vi "Target.vi"() -> ()   [LabVIEW 2025]
uses:
  <vilib>/Platform/TimedLoop/XDataNode/timing_clust.ctl
  <vilib>/Platform/TimedLoop/XDataNode/nitl_modes.ctl
  <vilib>/Platform/TimedLoop/XDataNode/wakeup.ctl
  <vilib>/rvi/Emulation/niFpgaSctlEmulationGetInTimedLoop.vi
  <vilib>/rvi/Emulation/niFpgaEmulationReportErrorSimple.vi
  <vilib>/rvi/Emulation/niFpgaGetClockAttributes.vi
  <vilib>/rvi/Emulation/niFpgaCriticalErrorInLSC.vi
  <vilib>/rvi/linearAlgebra/MatrixMultiply/simVIs/SubVI/nifxpla_MatrixMultiply_SimMatrixSizes.vi
  <vilib>/rvi/linearAlgebra/MatrixMultiply/simVIs/SubVI/nifxpla_MatrixMultiply_Sim4WireAdapterVector.vi
  <vilib>/rvi/linearAlgebra/MatrixMultiply/simVIs/SubVI/nifxpla_MatrixMultiply_SimFrameHandShake.vi
  <vilib>/rvi/linearAlgebra/MatrixMultiply/simVIs/SubVI/nifxpla_MatrixMultiply_SimEndlessCounter.vi
  <vilib>/rvi/linearAlgebra/MatrixMultiply/simVIs/SubVI/nifxpla_MatrixMultiply_SimVectorDataBuffer.vi
  <vilib>/rvi/ClientSDK/Core/DevComputerLib/Private/Multiply(dfxp64).vi
  <vilib>/rvi/ClientSDK/Core/DevComputerLib/Private/Dfxp128ToDfxp256.vi
  <vilib>/rvi/ClientSDK/Core/DevComputerLib/Private/Add(dfxp256).vi
  <vilib>/rvi/ClientSDK/Core/DevComputerLib/Private/Subtract(dfxp256).vi
  <vilib>/rvi/ClientSDK/Core/DevComputerLib/Private/ToDfxp64(dfxp256).vi
  <vilib>/platform/TimedLoop/XDataNode/XDataNode.xnode
  <vilib>/rvi/linearAlgebra/MatrixMultiply/XNode/nifxpla_MatrixMultiply.xnode
  <vilib>/rvi/linearAlgebra/MatrixMultiply/simVIs/nifxpla_MatrixMultiply_SimTemplateEinEout.vi
  <vilib>/rvi/linearAlgebra/MatrixMultiply/simVIs/nifxpla_MatrixMultiply_SimTemplateEinVout.vi
  <vilib>/rvi/linearAlgebra/MatrixMultiply/simVIs/nifxpla_MatrixMultiply_SimTemplateVinEout.vi
  <vilib>/rvi/linearAlgebra/MatrixMultiply/simVIs/nifxpla_MatrixMultiply_SimTemplateVinVout.vi
  <vilib>/Platform/TimedLoop/XDataNode/XDNodeRunTimeDep.lvlib
panel:
  out "C3+B":fxp<+/-,33,17>[](array[numeric])
  out "C3":fxp<+/-,32,16>[](array[numeric])
  out "Cycle Count 3":i32
  out "C2+B":fxp<+/-,33,17>[](array[numeric])
  out "C2":fxp<+/-,32,16>[](array[numeric])
  out "Cycle Count 2":i32
  out "C1+B":fxp<+/-,33,17>[](array[numeric])
  out "C1":fxp<+/-,32,16>[](array[numeric])
  out "Cycle Count":i32
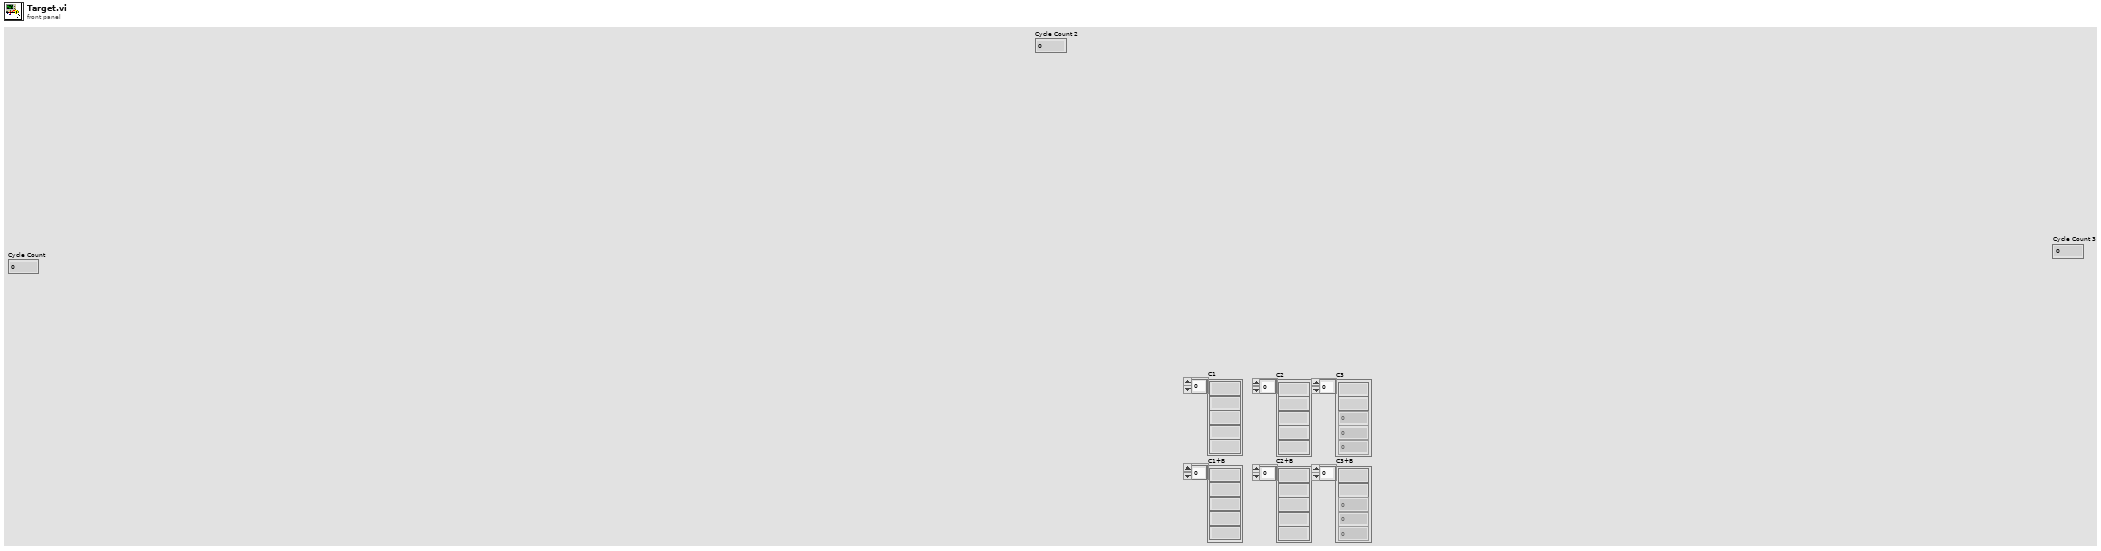
[diagram p1: front panel]
types:
  T1 = typedef "XDNodeRunTimeDep.lvlib/timing_clust.ctl" = cluster{"Expected End [f-1]":u64, "Actual End [f-1]":u64, "Finished Late? [f-1]":bool, "Expected End [i-1]":u64, "Actual End [i-1]":u64, "Finished Late? [i-1]":bool, "Expected Start [i]":u64, "Actual Start [i]":u64, "Expected Start [f]":u64, "Actual Start [f]":u64, "Source Name":string, "Structure Name":string, "Period":i64, "Deadline":i64, "Offset":i64, "Start":i64, "Priority":i32, "Timeout":i32, "Mode":T2, "Wakeup Reason":T3, "Error":errorcluster, "Source Type":string, "Secondary Source Type":string, "Global End Time":u64, "Global Start Time":u64, "Frame Duration":u64, "Iteration Duration":u64, "Assigned CPU":i32, "I/O Scan Engine Mode":u32}
  T2 = typedef "XDNodeRunTimeDep.lvlib/nitl_modes.ctl" = enum32{"No Change", "Process missed periods, maintain original phase", "Discard missed periods, maintain original phase", "Process missed periods, ignore original phase", "Discard missed periods, ignore original phase"}
  T3 = typedef "XDNodeRunTimeDep.lvlib/wakeup.ctl" = enum32{"Normal", "Aborted", "Asynchronous wakeup", "Timing source error", "Timed loop error", "Timeout"}
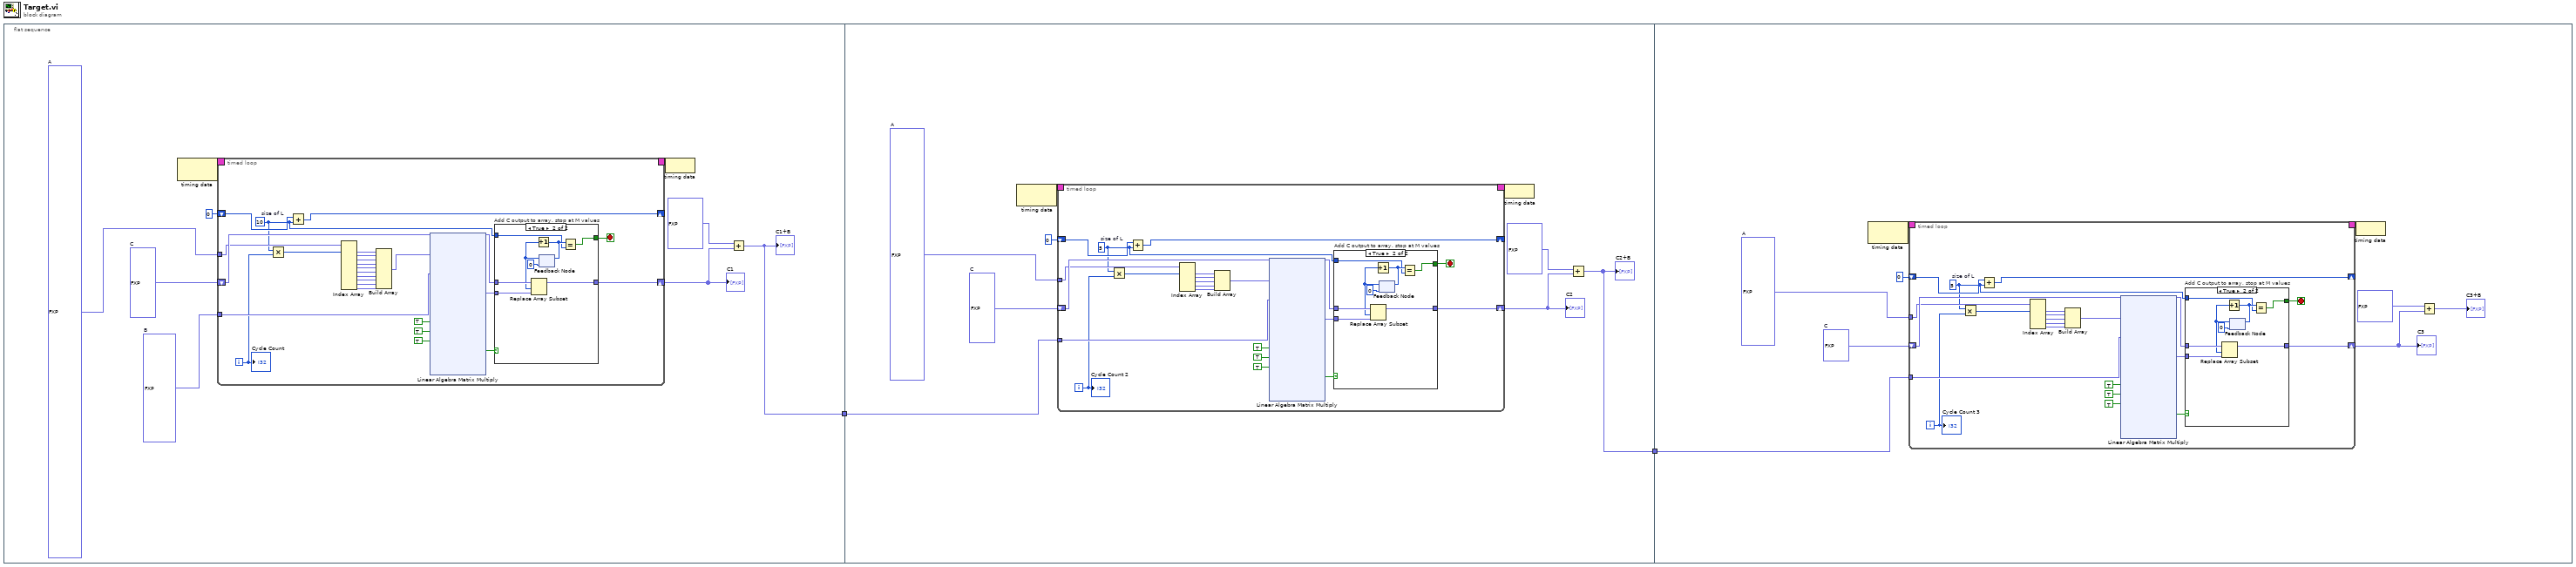
[diagram p0: block diagram]
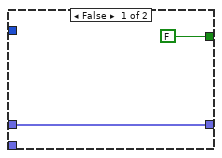
[diagram p2: hidden frame]
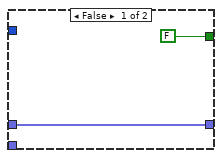
[diagram p3: hidden frame]
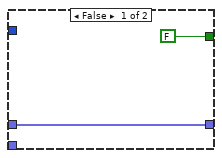
[diagram p4: hidden frame]
diagram:
  n1 = flat-sequence {
    tunnel: [w3] -> w2
    tunnel: w2 -> [w53]
    tunnel: [w52] -> w1
    tunnel: w1 -> [w96]
    frame #0 {
      w7 = fxp<+/-,32,16>[] [1.0, 2.0, 3.0, 4.0, 5.0, 1.0, 2.0, 3.0, 4.0, 5.0, 1.0, 2.0, 3.0, 4.0, 5.0, 1.0, 2.0, 3.0, 4.0, 5.0, 1.0, 2.0, 3.0, 4.0, 5.0, 1.0, 2.0, 3.0, 4.0, 5.0, 1.0, 2.0, 3.0, 4.0, 5.0, 1.0, 2.0, 3.0, 4.0, 5.0, 1.0, 2.0, 3.0, 4.0, 5.0, 1.0, 2.0, 3.0, 4.0, 5.0]  # A
      w8 = fxp<+/-,32,16>[] [1.0, 2.0, 3.0, 4.0, 5.0, 1.0, 2.0, 3.0, 4.0, 5.0]  # B
      w9 = fxp<+/-,32,16>[] [0.0, 0.0, 0.0, 0.0, 0.0]  # C
      n2 = node-c288() -> (w11:T1)  [unwired: 1 in]
      n3 = timed-loop {
        timing: w11 -> [_]
        timing-out: [_] -> w10
        shift-right: [w36] -> w5
        shift-left: w9 -> [w35]
        tunnel: w8 -> [w32]
        tunnel: w7 -> [w15]
        shift-right: [w28] -> _
        shift-left: 0 ("length") -> [w29]
        i -> [w14]
        stop <- w34 stop-if-true
        w13 = 10  # size of L
        n4 = Multiply(x=w13, y=w14) -> (x*y=w26:i32)
        n5 = Add(x=w29, y=w13) -> (x+y=w28:i32)
        n6 = Index Array(array=w15, index #1=w26) -> (element #1=w25:fxp<+/-,32,16>, element #2=w24:fxp<+/-,32,16>, element #3=w23:fxp<+/-,32,16>, element #4=w22:fxp<+/-,32,16>, element #5=w21:fxp<+/-,32,16>, element #6=w20:fxp<+/-,32,16>, element #7=w19:fxp<+/-,32,16>, element #8=w18:fxp<+/-,32,16>, element #9=w17:fxp<+/-,32,16>, element #10=w16:fxp<+/-,32,16>)  [unwired: 9 in]
        n7 = Build Array(w25, w24, w23, w22, w21, w20, w19, w18, w17, w16) -> (w12:fxp<+/-,32,16>[])
        n8 = xnode ("Linear Algebra Matrix Multiply")("ar"=w12, "br"=w32, "a valid"=TRUE, "b valid"=TRUE, "ready for output (T)"=TRUE) -> ("cr"=w31:fxp<+/-,64,36>[], "output valid"=w27:bool)  [unwired: 2 in, 4 out]
        n9 = case "Add C output to array, stop at M values" shown="True" w27 {
          tunnel: w31 -> [_ w43]
          tunnel: [w39 w46] -> w36
          tunnel: w35 -> [w39 w47]
          tunnel: [FALSE w44] -> w34
          tunnel: w13 -> [_ w40]
          frame False {
          }
          frame True {
            n10 = feedback #1(0 ("x")) -> (w42:i32)
            n11 = Replace Array Subset(array=w47, new element=w43, index=w42) -> (w46:fxp<+/-,32,16>[])
            n12 = Increment(x=w42) -> (x+1=w41:i32)
            n13 = feedback-in #1(w41) -> ()
            n14 = Equal?(x=w41, y=w40) -> (x = y?=w44:bool)
          }
        }
        "Cycle Count" <- w14
      }
      "C1" <- w5
      n15 = node-c288(w10) -> ()
      n16 = Add(x=fxp<+/-,32,16>[] [0.5, 0.5, 0.5, 0.5, 0.5], y=w5) -> (x+y=w3:fxp<+/-,33,17>[])
      "C1+B" <- w3
    }
    frame #1 {
      w57 = fxp<+/-,32,16>[] [1.0, 2.0, 3.0, 4.0, 5.0, 1.0, 2.0, 3.0, 4.0, 5.0, 1.0, 2.0, 3.0, 4.0, 5.0, 1.0, 2.0, 3.0, 4.0, 5.0, 1.0, 2.0, 3.0, 4.0, 5.0]  # A
      w58 = fxp<+/-,32,16>[] [0.0, 0.0, 0.0, 0.0, 0.0]  # C
      n17 = node-c288() -> (w60:T1)  [unwired: 1 in]
      n18 = timed-loop {
        timing: w60 -> [_]
        timing-out: [_] -> w59
        shift-right: [w80] -> w55
        shift-left: w58 -> [w79]
        tunnel: w53 -> [w76]
        tunnel: w57 -> [w64]
        shift-right: [w72] -> _
        shift-left: 0 ("length") -> [w73]
        i -> [w63]
        stop <- w78 stop-if-true
        w62 = 5  # size of L
        n19 = Multiply(x=w62, y=w63) -> (x*y=w70:i32)
        n20 = Add(x=w73, y=w62) -> (x+y=w72:i32)
        n21 = Index Array(array=w64, index #1=w70) -> (element #1=w69:fxp<+/-,32,16>, element #2=w68:fxp<+/-,32,16>, element #3=w67:fxp<+/-,32,16>, element #4=w66:fxp<+/-,32,16>, element #5=w65:fxp<+/-,32,16>)  [unwired: 4 in]
        n22 = Build Array(w69, w68, w67, w66, w65) -> (w61:fxp<+/-,32,16>[])
        n23 = xnode ("Linear Algebra Matrix Multiply")("ar"=w61, "br"=w76, "a valid"=TRUE, "b valid"=TRUE, "ready for output (T)"=TRUE) -> ("cr"=w75:fxp<+/-,64,36>[], "output valid"=w71:bool)  [unwired: 2 in, 4 out]
        n24 = case "Add C output to array, stop at M values" shown="True" w71 {
          tunnel: w75 -> [_ w87]
          tunnel: [w83 w90] -> w80
          tunnel: w79 -> [w83 w91]
          tunnel: [FALSE w88] -> w78
          tunnel: w62 -> [_ w84]
          frame False {
          }
          frame True {
            n25 = feedback #2(0 ("x")) -> (w86:i32)
            n26 = Replace Array Subset(array=w91, new element=w87, index=w86) -> (w90:fxp<+/-,32,16>[])
            n27 = Increment(x=w86) -> (x+1=w85:i32)
            n28 = feedback-in #2(w85) -> ()
            n29 = Equal?(x=w85, y=w84) -> (x = y?=w88:bool)
          }
        }
        "Cycle Count 2" <- w63
      }
      "C2" <- w55
      n30 = node-c288(w59) -> ()
      n31 = Add(x=fxp<+/-,32,16>[] [0.5, 0.5, 0.5, 0.5, 0.5], y=w55) -> (x+y=w52:fxp<+/-,33,17>[])
      "C2+B" <- w52
    }
    frame #2 {
      w101 = fxp<+/-,32,16>[] [2.0, 2.0, 2.0, 2.0, 2.0, 2.0, 2.0, 2.0, 2.0, 2.0]  # A
      w102 = fxp<+/-,32,16>[] [0.0, 0.0]  # C
      n32 = node-c288() -> (w104:T1)  [unwired: 1 in]
      n33 = timed-loop {
        timing: w104 -> [_]
        timing-out: [_] -> w103
        shift-right: [w124] -> w99
        shift-left: w102 -> [w123]
        tunnel: w96 -> [w120]
        tunnel: w101 -> [w108]
        shift-right: [w116] -> _
        shift-left: 0 ("length") -> [w117]
        i -> [w107]
        stop <- w122 stop-if-true
        w106 = 5  # size of L
        n34 = Multiply(x=w106, y=w107) -> (x*y=w114:i32)
        n35 = Add(x=w117, y=w106) -> (x+y=w116:i32)
        n36 = Index Array(array=w108, index #1=w114) -> (element #1=w113:fxp<+/-,32,16>, element #2=w112:fxp<+/-,32,16>, element #3=w111:fxp<+/-,32,16>, element #4=w110:fxp<+/-,32,16>, element #5=w109:fxp<+/-,32,16>)  [unwired: 4 in]
        n37 = Build Array(w113, w112, w111, w110, w109) -> (w105:fxp<+/-,32,16>[])
        n38 = xnode ("Linear Algebra Matrix Multiply")("ar"=w105, "br"=w120, "a valid"=TRUE, "b valid"=TRUE, "ready for output (T)"=TRUE) -> ("cr"=w119:fxp<+/-,64,36>[], "output valid"=w115:bool)  [unwired: 2 in, 4 out]
        n39 = case "Add C output to array, stop at M values" shown="True" w115 {
          tunnel: w119 -> [_ w131]
          tunnel: [w127 w134] -> w124
          tunnel: w123 -> [w127 w135]
          tunnel: [FALSE w132] -> w122
          tunnel: w106 -> [_ w128]
          frame False {
          }
          frame True {
            n40 = feedback #3(0 ("x")) -> (w130:i32)
            n41 = Replace Array Subset(array=w135, new element=w131, index=w130) -> (w134:fxp<+/-,32,16>[])
            n42 = Increment(x=w130) -> (x+1=w129:i32)
            n43 = feedback-in #3(w129) -> ()
            n44 = Equal?(x=w129, y=w128) -> (x = y?=w132:bool)
          }
        }
        "Cycle Count 3" <- w107
      }
      "C3" <- w99
      n45 = node-c288(w103) -> ()
      n46 = Add(x=fxp<+/-,32,16>[] [0.5, 0.5], y=w99) -> (x+y=→"C3+B":fxp<+/-,33,17>[])
    }
  }
